vi "Write.vi"(10 "Double Array":dbl[](array[numeric]), 11 "Double Array in":refnum<class "Double Array.lvclass">) -> (3 "Double Array out":refnum<class "Double Array.lvclass">)   [LabVIEW 2020, in "Data.lvlib" / "Double Array.lvclass"]
doc: "Write U32 Array."
uses:
  Double Array.lvclass
  Double Array.lvclass/Double Array.ctl
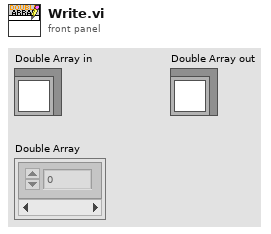
[diagram p1: front panel]
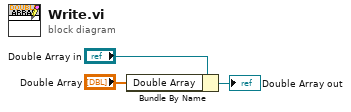
[diagram p0: block diagram]
diagram:
  n1 = Bundle By Name(cluster="Double Array in", "Double Array"="Double Array") -> (→"Double Array out":refnum<class "Double Array.lvclass">)
